vi "Problem5GraphGen.vi"() -> ()   [LabVIEW 2014]
uses:
  <vilib>/measure/NI_MABase.lvlib
panel:
  in  "sampling info":cluster{"Fs":dbl, "#s":dbl}={"Fs"=1000.0, "#s"=1000.0} {"Fs" format="%.2p"}
  in  "tones":T1(array[cluster])=[{"frequency"=100.0, "amplitude"=1.0, "phase"=0.0}, {"frequency"=22500.0, "amplitude"=0.1, "phase"=0.0}] {"phase" format="%.2p"; "amplitude" format="%0.2p"; "frequency" format="%0.2p"}
  out "Waveform Graph":waveform(dbl)(graph)
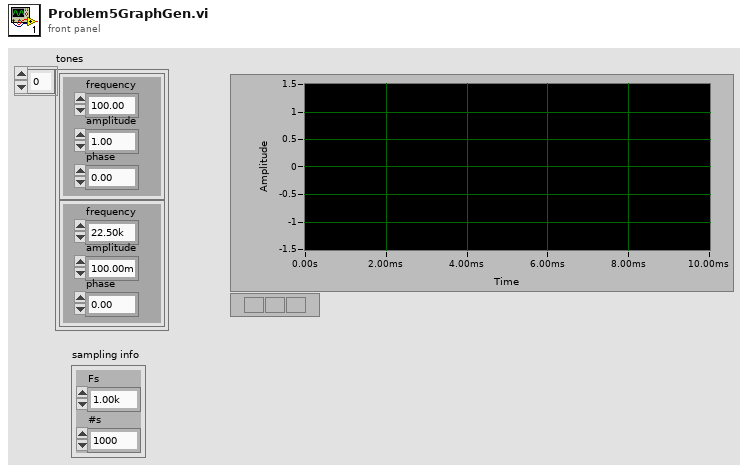
[diagram p1: front panel]
types:
  T1 = cluster{"frequency":dbl, "amplitude":dbl, "phase":dbl}[]
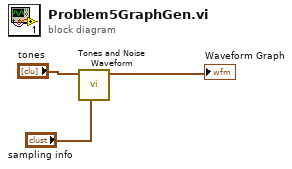
[diagram p0: block diagram]
diagram:
  n1 = call <vilib>:"Tones and Noise Waveform.vi"("sampling info"="sampling info", "tones"="tones") -> ("signal out"=→"Waveform Graph":waveform(dbl))  [unwired: 8 in, 1 out]
